vi "GPS - Standalone Main.vi"() -> ()   [LabVIEW 2021]
uses:
  <vilib>/Platform/TimedLoop/XDataNode/timing_clust.ctl
  <vilib>/Platform/TimedLoop/XDataNode/nitl_modes.ctl
  <vilib>/Platform/TimedLoop/XDataNode/wakeup.ctl
  <vilib>/platform/TimedLoop/XDataNode/XDataNode.xnode
  <vilib>/Platform/TimedLoop/XDataNode/XDNodeRunTimeDep.lvlib
panel:
  out "error out 2":errorcluster
  in  "error in (no error) 2":errorcluster
  out "VISA Refnum out":refnum<visa-resource-name>
  out "XY Graph":cluster{dbl[], dbl[]}(graph)
  out "Long":dbl[](array[numeric])
  out "Lat":dbl[](array[numeric])
  out "GNRMC String Array":string[](array[string])
  in  "stop":bool
  out "Longitude W (deg)":dbl
  out "Latitude N (deg)":dbl
  out "error out":errorcluster
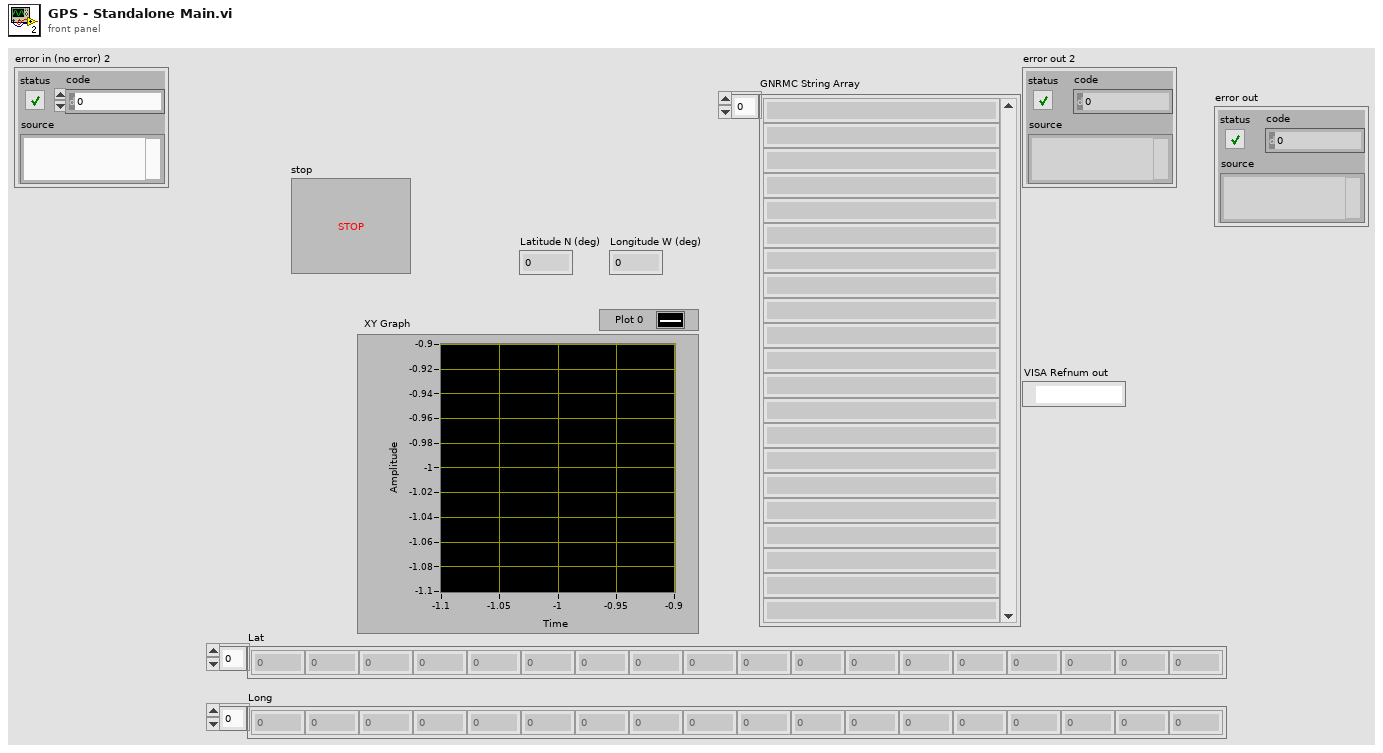
[diagram p1: front panel]
types:
  T1 = typedef "XDNodeRunTimeDep.lvlib/timing_clust.ctl" = cluster{"Expected End [f-1]":u64, "Actual End [f-1]":u64, "Finished Late? [f-1]":bool, "Expected End [i-1]":u64, "Actual End [i-1]":u64, "Finished Late? [i-1]":bool, "Expected Start [i]":u64, "Actual Start [i]":u64, "Expected Start [f]":u64, "Actual Start [f]":u64, "Source Name":string, "Structure Name":string, "Period":i64, "Deadline":i64, "Offset":i64, "Start":i64, "Priority":i32, "Timeout":i32, "Mode":T2, "Wakeup Reason":T3, "Error":errorcluster, "Source Type":string, "Secondary Source Type":string, "Global End Time":u64, "Global Start Time":u64, "Frame Duration":u64, "Iteration Duration":u64, "Assigned CPU":i32, "I/O Scan Engine Mode":u32}
  T2 = typedef "XDNodeRunTimeDep.lvlib/nitl_modes.ctl" = enum32{"No Change", "Process missed periods, maintain original phase", "Discard missed periods, maintain original phase", "Process missed periods, ignore original phase", "Discard missed periods, ignore original phase"}
  T3 = typedef "XDNodeRunTimeDep.lvlib/wakeup.ctl" = enum32{"Normal", "Aborted", "Asynchronous wakeup", "Timing source error", "Timed loop error", "Timeout"}
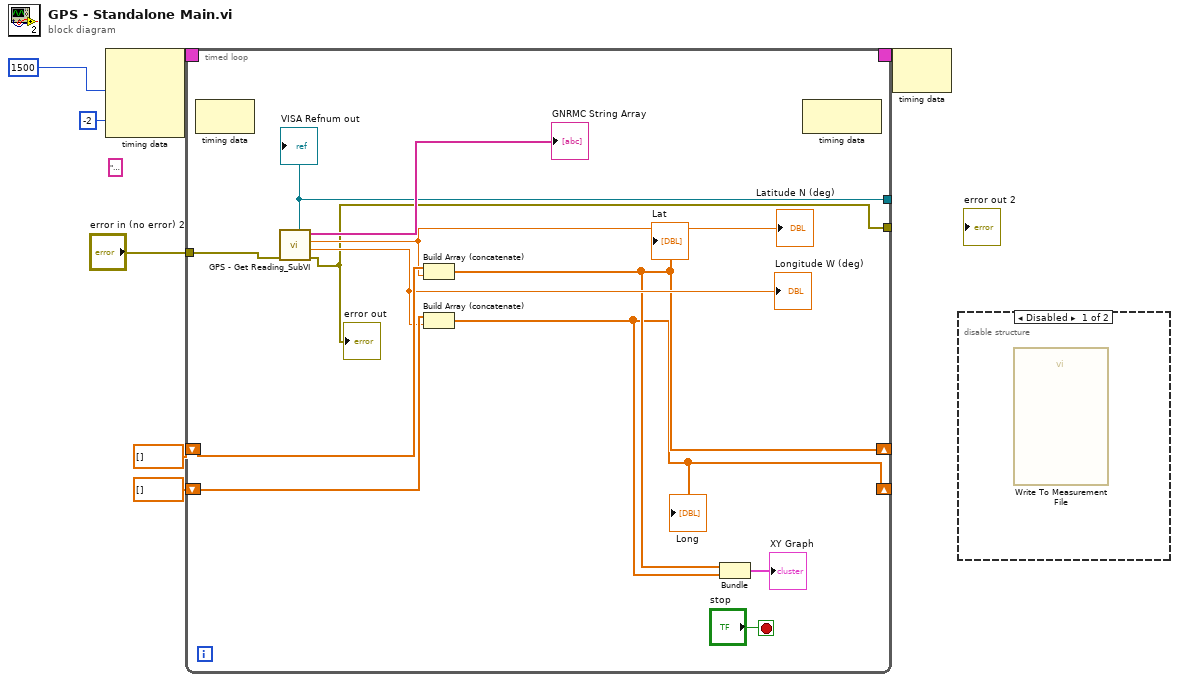
[diagram p0: block diagram]
diagram:
  (unwired) "14830.00,A,A*69\r\n$GNRMC,214831.00,A,3346.62967,N,08423.86388,W,0.022,,280324,,,A,V*0A\r\n$GNVTG,,T,,M,0.022,N,0.041,K,A*38\r\n$GNGGA,214831.00,3346.62967,N,08423.86388,W,1,12,0.68,298.4,M,-31.2,M,,*74\r\n$GNGSA,A,3,05,06,11,12,19,20,22,25,,,,,1.36,0.68,1.17,1*01\r\n$GNGSA,A,3,24,25,,,,,,,,,,,1.36,0.68,1.17,3*0F\r\n$GNGSA,A,3,19,24,26,29,44,45,22,,,,,,1.36,0.68,1.17,4*09\r\n$GNGSA,A,3,,,,,,,,,,,,,1.36,0.68,1.17,5*08\r\n$GPGSV,3,1,11,05,26,205,26,06,46,038,29,09,15,076,24,11,67,330,30,1*68\r\n$GPGSV,3,2,11,12,51,290,28,17,17,109,26,19,39,097,32,20,63,200,36,1*62\r\n$GPGSV,3,3,11,22,10,160,17,24,00,234,06,25,25,312,27,1*54\r\n$GPGSV,1,1,03,04,01,041,,44,38,229,,46,29,241,,0*5A\r\n$GAGSV,1,1,03,04,17,104,26,24,25,170,22,25,61,230,34,7*42\r\n$GAGSV,2,1,07,10,39,045,,11,60,014,,12,17,057,,18,43,309,,0*7A\r\n$GAGSV,2,2,07,18,43,309,,19,06,049,,34,02,254,,0*42\r\n$GBGSV,2,1,07,19,47,102,36,22,28,168,22,24,21,292,28,26,27,238,23,1*75\r\n$GBGSV,2,2,07,29,28,082,22,44,32,300,28,45,07,188,20,1*47\r\n$GQGSV,1,1,00,0*64\r\n$GNGLL,3346.62967,N,08423.86388,W,214831.00,A,A*66\r\n$GNRMC,214832.00,A,3346.62971,N,08423.86383,W,0.129,,280324,,,A,V*0F\r\n$GNVTG,,T,,M,0.129,N,0.238,K,A*3E\r\n$GNGGA,214832.00,3346.62971,N,08423.86383,W,1,12,0.68,298.3,M,-31.2,M,,*7C\r\n$GNGSA,A,3,05,06,11,12,19,20,22,25,,,,,1.36,0.68,1.17,1*01\r\n$GNGSA,A,3,24,25,,,,,,,,,,,1.36,0.68,1.17,3*0F\r\n$GNGSA,A,3,19,24,26,29,44,45,22,,,,,,1.36,0.68,1.17,4*09\r\n$GNGSA,A,3,,,,,,,,,,,,,1.36,0.68,1.17,5*08\r\n$GPGSV,3,1,11,05,26,205,27,06,46,038,28,09,15,076,26,11,67,330,32,1*68\r\n$GPGSV,3,2,11,12,51,290,33,17,17,109,27,19,39,097,33,20,63,200,33,1*6D\r\n$GPGSV,3,3,11,22,10,160,14,24,00,234,06,25,25,312,25,1*55\r\n$GPGSV,1,1,03,04,01,041,,44,38,229,,46,29,241,,0*5A\r\n$GAGSV,1,1,03,04,17,104,26,24,25,170,23,25,61,230,35,7*42\r\n$GAGSV,2,1,07,10,39,045,,11,60,014,,12,17,057,,18,43,309,,0*7A\r\n$GAGSV,2,2,07,18,43,309,,19,06,049,,34,02,254,,0*42" ("delimiter (Tab)")
  n1 = node-c288(i64 1500 ("Period"), -2 ("Processor")) -> (w7:T1)  [unwired: 2 in]
  n2 = timed-loop {
    timing: w7 -> [_]
    timing-out: [_] -> w6
    shift-right: [w13] -> _
    shift-left: dbl[] [] ("y") -> [w19]
    shift-right: [w12] -> _
    shift-left: dbl[] [] ("y") -> [w17]
    tunnel: "error in (no error) 2" -> [w10]
    tunnel: [w9] -> _
    tunnel: [w8] -> _
    stop <- "stop" stop-if-true
    n3 = node-c288() -> ()  [unwired: 1 in, 1 out]
    n4 = call "GPS - Get Reading_SubVI.vi"("error in (no error) 2"=w10) -> ("error out"=w8:errorcluster, "Longitude W (deg)"=w16:dbl, "Latitude N (deg)"=w18:dbl, "GNRMC String Array"=→"GNRMC String Array":string[], "VISA resource name out"=w9:refnum<visa-resource-name>)  [unwired: 6 in]
    "error out" <- w8
    "Latitude N (deg)" <- w18
    "Longitude W (deg)" <- w16
    "VISA Refnum out" <- w9
    n5 = Build Array (concatenate)(w19, w18) -> (w13:dbl[])
    "Lat" <- w13
    n6 = Build Array (concatenate)(w17, w16) -> (w12:dbl[])
    "Long" <- w12
    n7 = Bundle(w13, w12) -> (→"XY Graph":cluster{dbl[], dbl[]})  [unwired: 1 in]
    n8 = node-c288() -> ()  [unwired: 1 in, 1 out]
  }
  n9 = node-c288(w6) -> ()  [unwired: 1 out]
  n10 = disable-structure shown="Disabled" {
    frame Disabled {
      n11 = call "Write To Measurement File"() -> ()  [unwired: 17 in, 3 out]
    }
    frame Enabled {
    }
  }
